vi "Config.vi"(8 "error in (no error)":errorcluster, 10 "Setting":variant, 11 "Sim Scope in":refnum<class "Sim Scope.lvclass">) -> (0 "error out":errorcluster, 3 "Sim Scope out":refnum<class "Sim Scope.lvclass">)   [LabVIEW 2025, in "Scope.lvlib" / "Sim Scope.lvclass"]
uses:
  Sim Scope.lvclass
  C:/Users/Public/Documents/Sandia National Labs/TSS Plugin/CEF.lvlibp/Node/CEF_Node.lvclass
  C:/Users/Public/Documents/Sandia National Labs/TSS Plugin/Abstract Engine.lvlibp/Abstract Instrument/Abstract Instrument.lvclass
  Scope Channel/Scope Channel.lvclass
  Users/Public/Documents/Sandia National Labs/TSS Plugin/Abstract Engine.lvlibp/Abstract Instrument/Channel.ctl
  Scope Channel configuration/Scope Channel configuration.lvclass
  C:/Users/Public/Documents/Sandia National Labs/TSS Plugin/Abstract Engine.lvlibp/Channel configuration/Channel configuration.lvclass
  Users/Public/Documents/Sandia National Labs/TSS Plugin/CEF.lvlibp/Node/ReadChildren.vi
  Users/Public/Documents/Sandia National Labs/TSS Plugin/Abstract Engine.lvlibp/Channel configuration/Read Channel Setting.vi
  Users/Public/Documents/Sandia National Labs/TSS Plugin/CEF.lvlibp/Node/CEF_Node.lvclass
  Users/Public/Documents/Sandia National Labs/TSS Plugin/CEF.lvlibp/serializable configuration/CEF_serializable configuration.lvclass
  Users/Public/Documents/Sandia National Labs/TSS Plugin/Abstract Engine.lvlibp/Abstract Instrument/Abstract Instrument.lvclass
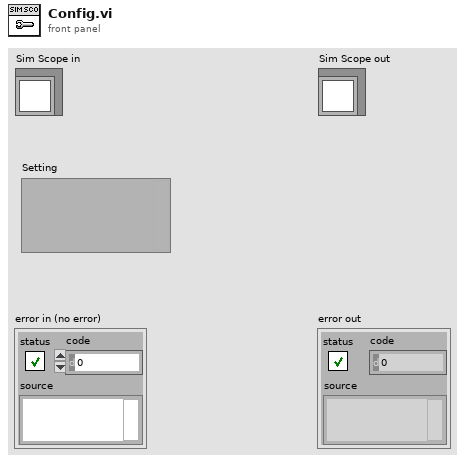
[diagram p1: front panel]
types:
  T1 = typedef "Abstract Engine.lvlibp/Abstract Instrument.lvclass/Channel.ctl" = cluster{"Alias":string, "DataType":enum16{"Anaolg Input", "Waveform"}, "Unit":enum16{"---", "V", "A", "Ohm", "Hz", "uF", "degC", "deg"}, "Upper limit":dbl, "Lower limit":dbl, "Measurement":variant}
  T2 = typedef "Abstract Engine.lvlibp/Channel configuration.lvclass/Default Channel.ctl" = cluster{"Address":string, "SW Alias":string, "Enabled":bool, "Type":string, "Description":string}
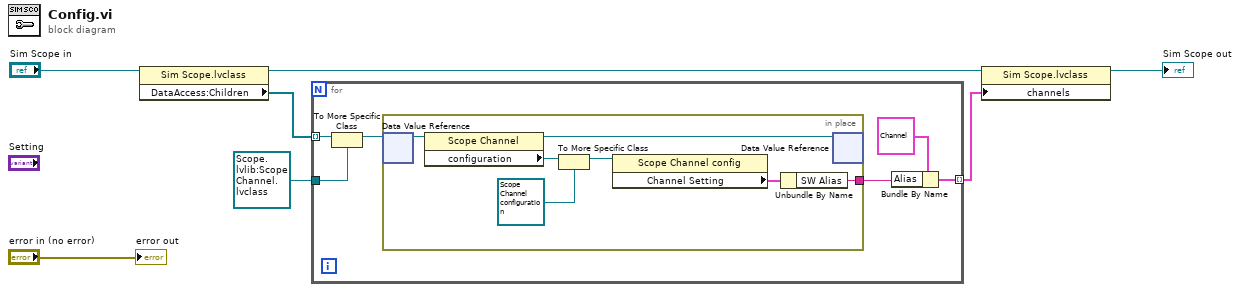
[diagram p0: block diagram]
diagram:
  n1 = property class="Sim Scope.lvclass"(reference="Sim Scope in") -> (reference out=w5:refnum<class "Sim Scope.lvclass">, "DataAccess:Children"=w7:refnum<data-value>[])  [unwired: 1 in, 1 out]
  n2 = for {
    tunnel: w7 -> [w12] mode=indexing
    tunnel: refnum<data-value> refnum ("data value reference") -> [w11]
    tunnel: [w9] -> w1 mode=indexing
    n3 = To More Specific Class(target class=w11, reference=w12) -> (specific class reference=w13:refnum<data-value>)  [unwired: 1 in, 1 out]
    n4 = in-place {
      in-place-border: [w14] -> w10
      # "Initialize the front panel controls when loaded"
      n5 = in-place-dvr #1(w13) -> (w20:refnum<class "Scope Channel.lvclass">)  [unwired: 1 out]
      n6 = property class="Scope Channel"(reference=w20) -> (reference out=w19:refnum<class "Scope Channel.lvclass">, "configuration"=w18:refnum<class "CEF_serializable configuration.lvclass">)  [unwired: 1 in, 1 out]
      n7 = To More Specific Class(target class=refnum<class "Scope Channel configuration.lvclass"> refnum ("Scope.lvlib:Scope Channel configuration.lvclass"), reference=w18) -> (specific class reference=w17:refnum<class "Scope Channel configuration.lvclass">)  [unwired: 1 in, 1 out]
      n8 = property class="Scope Channel config"(reference=w17) -> ("Channel Setting"=w15:T2)  [unwired: 1 in, 2 out]
      n9 = Unbundle By Name(w15) -> ("SW Alias"=w14:string)
      n10 = in-place-dvr #1(w19) -> ()  [unwired: 2 out]
    }
    n11 = Bundle By Name(cluster=T1 {"Alias"="ch0", "DataType"=enum."Anaolg Input", "Unit"=enum."V", "Upper limit"=10.0, "Lower limit"=-10.0, "Measurement"=variant} ("Channel"), "Alias"=w10) -> (w9:T1)
  }
  n12 = property class="Sim Scope.lvclass"(reference=w5, "channels"=w1) -> (reference out=→"Sim Scope out":refnum<class "Sim Scope.lvclass">)  [unwired: 1 in, 1 out]
  "error out" <- "error in (no error)"
